vi "Pass If State Configurations Match.vi"(8 "error in (no error)":errorcluster, 9 "Known State Configurations":T1, 10 "Imported State Configurations":T1, 11 "Test Case in":refnum<class "Routing and Faulting Import Unit Tests.lvclass">) -> (0 "error out":errorcluster, 3 "Test Case out":refnum<class "Routing and Faulting Import Unit Tests.lvclass">)   [LabVIEW 2017, in "Routing and Faulting Import Unit Tests.lvclass"]
uses:
  Routing and Faulting Import Unit Tests.lvclass
  Shared/Channel States.ctl
  Shared/Routing State.ctl
  Shared/Connection.ctl
  Shared/Routing and Faulting Shared.lvlib
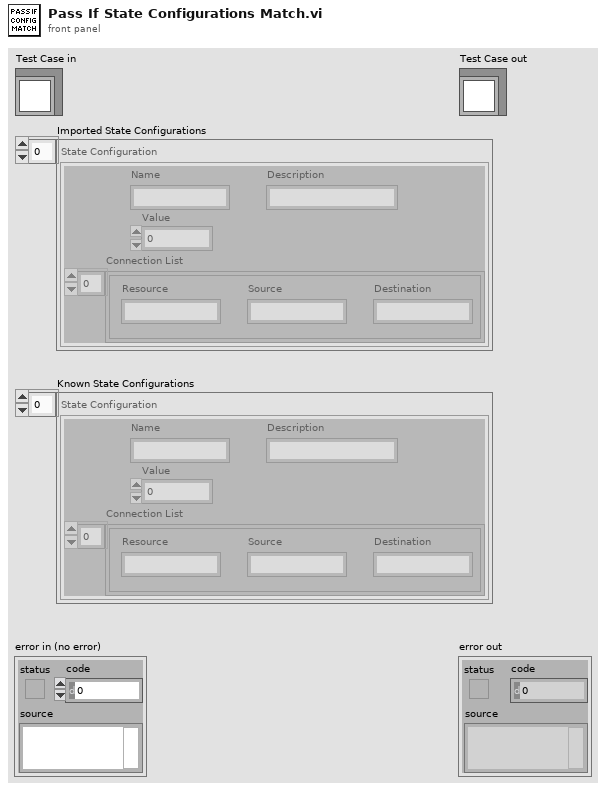
[diagram p1: front panel]
types:
  T1 = typedef "Routing and Faulting Shared.lvlib/Channel States.ctl" = T2[]
  T2 = typedef "Routing and Faulting Shared.lvlib/Routing State.ctl" = cluster{"Name":string, "Description":string, "Value":i32, "Connection List":T3[]}
  T3 = typedef "Routing and Faulting Shared.lvlib/Connection.ctl" = cluster{"Resource":string, "Source":string, "Destination":string}
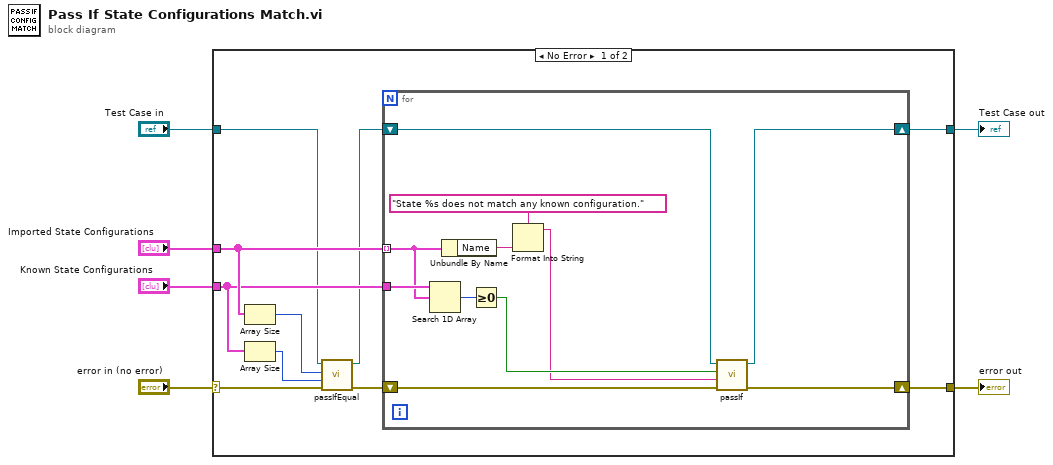
[diagram p0: block diagram]
diagram:
  n1 = case shown="No Error" "error in (no error)" {
    selector: "error in (no error)" -> [w16 w29]
    tunnel: [w10 w29] -> w5
    tunnel: [w9 w28] -> w3
    tunnel: "Test Case in" -> [w8 w28]
    tunnel: "Imported State Configurations" -> [w12 _]
    tunnel: "Known State Configurations" -> [w11 _]
    frame No Error {
      n2 = Array Size(array=w12) -> (size(s)=w14:i32)
      n3 = Array Size(array=w11) -> (size(s)=w15:i32)
      n4 = call-dynamic "passIfEqual.vi"("error in (no error)"=w16, "y"=w15, "x"=w14, "TestCase in"=w8) -> ("error out"=w13:errorcluster, "TestCase out"=w7:refnum<class "Routing and Faulting Import Unit Tests.lvclass">)  [unwired: 6 in]
      n5 = for {
        shift-right: [w20] -> w10
        shift-left: w13 -> [w25]
        tunnel: w12 -> [w23] mode=indexing
        tunnel: w11 -> [w27]
        shift-right: [w17] -> w9
        shift-left: w7 -> [w18]
        n6 = Search 1D Array(1D array=w27, element=w23) -> (index of element=w26:i32)  [unwired: 1 in]
        n7 = Unbundle By Name(w23) -> ("Name"=w21:string)
        n8 = Greater Or Equal To 0?(x=w26) -> (x >= 0?=w24:bool)
        n9 = Format Into String(format string="State %s does not match any known configuration." ("message (\"\")"), w21) -> (resulting string=w19:string)  [unwired: 2 in, 1 out]
        n10 = call-dynamic "passIf.vi"("error in (no error)"=w25, "message (\"\")"=w19, "pass"=w24, "TestCase in"=w18) -> ("error out"=w20:errorcluster, "TestCase out"=w17:refnum<class "Routing and Faulting Import Unit Tests.lvclass">)  [unwired: 6 in]
      }
    }
    frame Error {
    }
  }
  "error out" <- w5
  "Test Case out" <- w3
